vi "Parse Response JSON.vi"(8 "error in (no error)":errorcluster, 10 "Response JSON":string, 11 "RGetInputList in":refnum<class "RGetInputList.lvclass">) -> (0 "error out":errorcluster, 3 "RGetInputList out":refnum<class "RGetInputList.lvclass">)   [LabVIEW 2020, in "obs-websocket.lvlib" / "RGetInputList.lvclass"]
uses:
  RGetInputList.lvclass
  Input.ctl
  Input Settings.ctl
  RGetInputList.lvclass/RGetInputList.ctl
  <vilib>/IlluminatedG/lv-web-crypto/lv-json/JSON/JSON.lvlib
  obs-websocket.lvlib
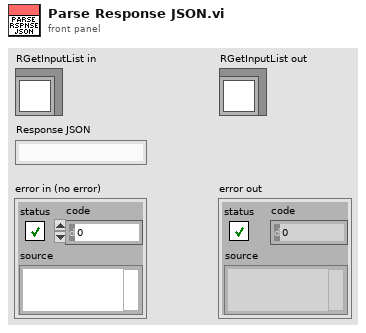
[diagram p1: front panel]
types:
  T1 = typedef "JSON.lvlib/JSON Item Type.ctl" = enum16{"unknown", "null", "Array", "Object", "String", "Number", "Boolean"}
  T2 = typedef "obs-websocket.lvlib/Input.ctl" = cluster{"Kind":string, "Name":string, "Unversioned Kind":string, "Input Settings":T3}
  T3 = typedef "obs-websocket.lvlib/Input Settings.ctl" = cluster{"Deactive When Not Showing":bool, "Frame Interval":i32, "Last Resolution":string, "Last Video Device ID":string, "Res Type":i32, "Resolution":string, "Video Device ID":string}
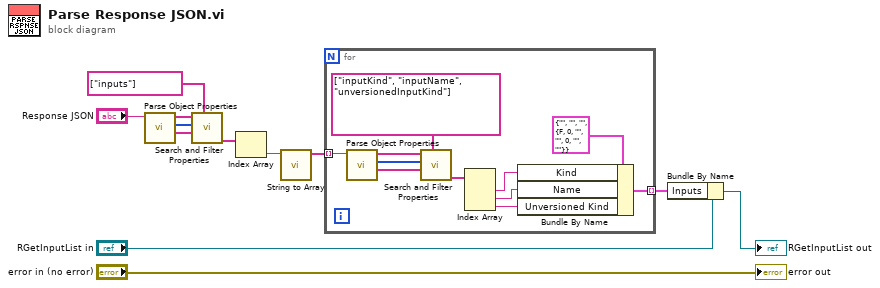
[diagram p0: block diagram]
diagram:
  n1 = call <vilib>:"Parse Object Properties.vi"("JSON String"="Response JSON") -> ("Values"=w8:string[], "Item Types"=w9:T1[], "Keys"=w10:string[])  [unwired: 7 in, 1 out]
  n2 = call <vilib>:"Search and Filter Properties.vi"("Search Keys"=string[] ["inputs"], "Values In"=w8, "Types In"=w9, "Keys In"=w10) -> ("Filtered Values"=w6:string[])  [unwired: 1 in, 6 out]
  n3 = Index Array(array=w6) -> (element=w5:string)  [unwired: 1 in]
  n4 = call <vilib>:"String to Array.vi"("Array String In"=w5) -> ("JSON Strings"=w4:string[])  [unwired: 10 in]
  n5 = for {
    tunnel: w4 -> [w23] mode=indexing
    tunnel: [w13] -> w3 mode=indexing
    n6 = call <vilib>:"Parse Object Properties.vi"("JSON String"=w23) -> ("Values"=w20:string[], "Item Types"=w21:T1[], "Keys"=w22:string[])  [unwired: 7 in, 1 out]
    n7 = call <vilib>:"Search and Filter Properties.vi"("Search Keys"=string[] ["inputKind", "inputName", "unversionedInputKind"], "Values In"=w20, "Types In"=w21, "Keys In"=w22) -> ("Filtered Values"=w18:string[])  [unwired: 1 in, 6 out]
    n8 = Index Array(array=w18) -> (element #1=w14:string, element #2=w15:string, element #3=w16:string)  [unwired: 3 in]
    n9 = Bundle By Name(cluster=T2 {"Kind"="", "Name"="", "Unversioned Kind"="", "Input Settings"={"Deactive When Not Showing"=FALSE, "Frame Interval"=0, "Last Resolution"="", "Last Video Device ID"="", "Res Type"=0, "Resolution"="", "Video Device ID"=""}} ("Input"), "Kind"=w14, "Name"=w15, "Unversioned Kind"=w16) -> (w13:T2)
  }
  n10 = Bundle By Name(cluster="RGetInputList in", "Inputs"=w3) -> (→"RGetInputList out":refnum<class "RGetInputList.lvclass">)
  "error out" <- "error in (no error)"
